vi "Load_SetList_HistoryUpdate_v4.vi"(1 "New Element":string, 2 "History in":string[](array[string])=["", "", "", "", "", "", "", "", "", "", "", "", "", "", "", "", "", ""]) -> (0 "History Out":string[](array[string]))   [LabVIEW 2013]
doc: "This VI adds the \"New Element\" to the history, provided it is not already an element. Pre-existing duplicates are not removed."
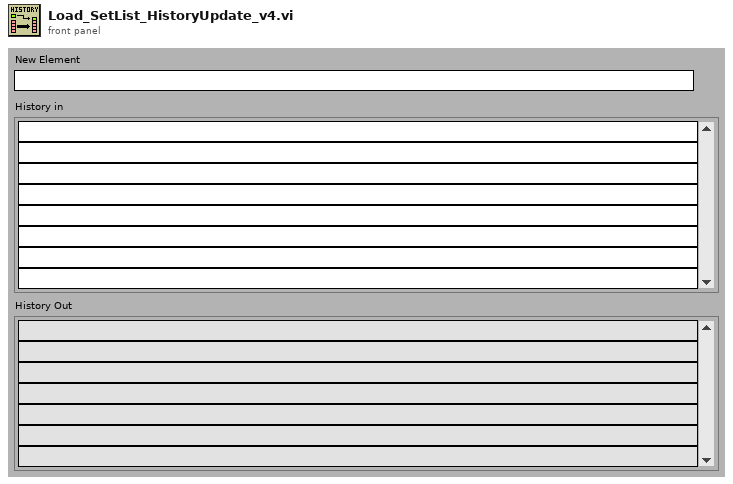
[diagram p1: front panel]
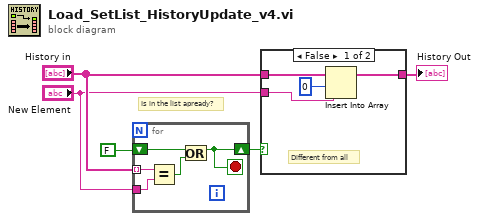
[diagram p0: block diagram]
diagram:
  # "Is in the list apready?"
  n1 = for {
    tunnel: "History in" -> [w10] mode=indexing
    tunnel: "New Element" -> [w9]
    shift-right: [w6] -> w3
    shift-left: FALSE -> [w7]
    stop <- w6 stop-if-true
    n2 = Equal?(x=w10, y=w9) -> (x = y?=w8:bool)
    n3 = Or(x=w7, y=w8) -> (x .or. y?=w6:bool)
  }
  n4 = case shown="False" w3 {
    tunnel: "History in" -> [w13 w15]
    tunnel: [w12 w15] -> w2
    tunnel: "New Element" -> [w11 _]
    frame False {
      # "Different from all"
      n5 = Insert Into Array(array=w13, index=0, new element=w11) -> (w12:string[])
    }
    frame True {
    }
  }
  "History Out" <- w2
